vi "Drag & Drop Run.vi"   [LabVIEW 2015]
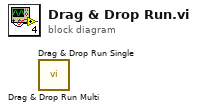
[diagram p0: block diagram]
diagram:
  n1 = call "Drag & Drop Run Multi.vi"() -> ()  [unwired: 8 in, 2 out]
  n2 = call "Drag & Drop Run Single.vi"() -> ()  [unwired: 8 in, 2 out]
